vi "Global_ACT_Data Out.vi"() -> ()   [LabVIEW 2023, in "Shooter FX_ACT.lvlib"]
uses:
  Shooter FX_ACT.lvlib
  Cluster_HW Output Values.ctl
  Shared Code/TypeDefs/Cluster_FX Sensor Values.ctl
  Shared Code/TypeDefs/Cluster_FX CloseLoop Values.ctl
  Shared Code/TypeDefs/Cluster_FX Current Values.ctl
  Shared Code/TypeDefs/Cluster_FX Voltage Values.ctl
  Cluster_SW Output Data.ctl
  ENUM_ACT_State.ctl
panel:
  out "ACT_Shooter_STATE":T1
  in  "ACT_Shooter_SW Output":T2
  out "ACT_Shooter_HW Output":T3
  in  "ACT_Shooter_CycleTime(S)":dbl
  # "The Names of the Data items in the Global Variable MUST describe who the Single Writer is\nFor Actuator Globals the the naming convention is\n   \nACT_Lib Name_Data Name\n\nExamples:\nACT_Drive_X axis\nACT_Hopper_AgitatorSpeed"
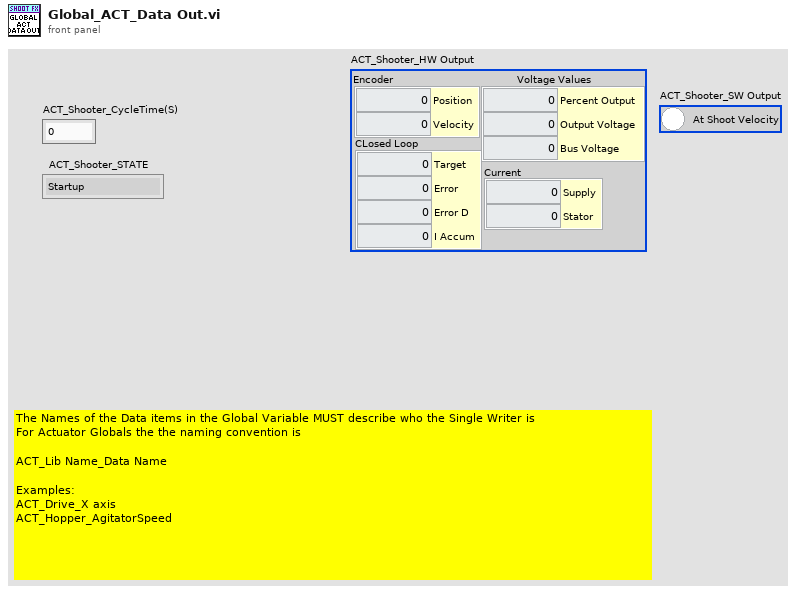
[diagram p1: front panel]
types:
  T1 = typedef "Shooter FX_ACT.lvlib/ENUM_ACT_State.ctl" = enum16{"Startup", "Configuring", "Stopping", "Moving Percent Out", "Moving to Position", "Shutdown"}
  T2 = typedef "Shooter FX_ACT.lvlib/Cluster_SW Output Data.ctl" = cluster{"At Shoot Velocity":bool}
  T3 = typedef "Shooter FX_ACT.lvlib/Cluster_HW Output Values.ctl" = cluster{"Encoder":T4, "Current":T5, "CLosed Loop":T6, "Voltage Values":T7}
  T4 = typedef "Cluster_FX Sensor Values.ctl" = cluster{"Position":i32, "Velocity":i32}
  T5 = typedef "Cluster_FX Current Values.ctl" = cluster{"Supply":dbl, "Stator":dbl}
  T6 = typedef "Cluster_FX CloseLoop Values.ctl" = cluster{"Target":dbl, "Error":i32, "Error D":dbl, "I Accum":dbl}
  T7 = typedef "Cluster_FX Voltage Values.ctl" = cluster{"Percent Output":dbl, "Output Voltage":dbl, "Bus Voltage":dbl}
diagram:
